vi "GlobalLongueurOnde.vi"() -> ()   [LabVIEW 2018]
panel:
  out "Numeric":dbl
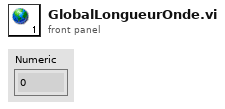
[diagram p1: front panel]
diagram:
